vi "PPMS Monitor and Control.vi"() -> ()   [LabVIEW 2019, in "instrument.PPMS.lvclass"]
doc: "This VI will launch the PPMS 2 Instrument backend that will contunously monitor the state of the instrument and log to the DSC. The user has the option of launching a user interface (default) or allowing the backend to run headless. Run \"Launch PPMS2 UI.vi\" here or on a different computer to have a remote user interface. You can also use the APIs like \"Get Temperturature\" interact programmatically with the PPMS 2 Instrument backend."
uses:
  instrument.PPMS/instrument.PPMS.lvclass
  <vilib>/JKI/JKI SMO/SMO/Typedefs/SMOState --Enum.ctl
  <vilib>/JKI/JKI SMO/SMO.UI/Typedefs/SMO.UI State--enum.ctl
  C:/Program Files (x86)/National Instruments/LabVIEW 2019/user.lib/LevyLab/Instrument Framework/Instrument/Instrument.lvclass
  C:/Program Files (x86)/National Instruments/LabVIEW 2019/vi.lib/JKI/JKI SMO/SMO/SMO.lvclass
  instrument.PPMS UI/Instrument UI.PPMS.lvclass
  C:/Program Files (x86)/National Instruments/LabVIEW 2019/vi.lib/JKI/JKI SMO/SMO.UI/SMO.UI.lvclass
  C:/Program Files (x86)/National Instruments/LabVIEW 2019/user.lib/LevyLab/Instrument Framework/Instrument UI/Instrument UI.lvclass
  <userlib>/LevyLab/Configuration/Configuration.lvclass
  PPMS/Select PPMS--Enum.ctl
  <vilib>/Utility/sysdir.llb/System Directory Type.ctl
  <vilib>/JKI/JKI SMO/SMO/SMO.lvclass/SMO.ctl
  <vilib>/JKI/JKI SMO/SMO.UI/SMO.UI.lvclass/SMO.UI.ctl
  <vilib>/JKI/JKI SMO/SMO/Private/ReftoDVR--SMO.vi
  <vilib>/JKI/JKI SMO/SMO.UI/SMO.UI.ReftoDVR.vi
  <vilib>/JKI/JKI SMO/SMO/SMO.lvclass
  <vilib>/JKI/JKI SMO/SMO.UI/SMO.UI.lvclass
  <userlib>/LevyLab/Instrument Framework/Instrument UI/Instrument UI.lvclass
  PPMS/PPMS.lvlib
  <userlib>/LevyLab/Instrument Framework/Instrument/Instrument.lvclass
  <vilib>/Utility/config.llb/NI_LVConfig.lvlib
panel:
  in  "Examine Configuration.ini":bool
  out "version":string
  in  "Debug Mode":bool
  in  "Select PPMS":T1(ring) caption="Enum"
  in  "Stop Application":bool caption="Stop"
  in  "Start Application":bool caption="Play"
  in  "Splash Status":string="Push Start to Start..." caption="String"
  out "error out":errorcluster
  # "PPMS\nMonitor\n&\nControl"
  # "PPMS1: 130.49.180.18\nPPMS2: 130.49.180.87\nPPMS3: 130.49.180.47\nsimulate: localhost"
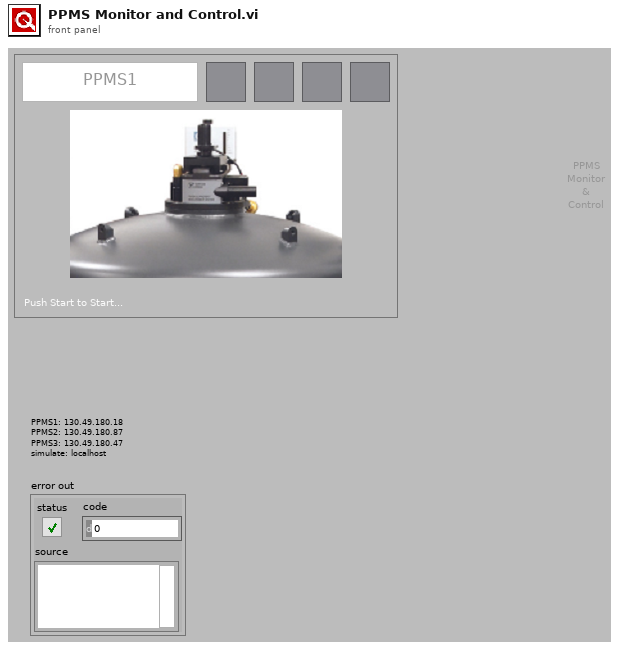
[diagram p1: front panel]
types:
  T1 = enum16{"PPMS1", "PPMS2", "PPMS3", "OptiCool", "PPMS-W-1", "Simulate PPMS", "Simulate DynaCool", "Simulate OptiCool"}
  T2 = typedef "SMO.lvclass/SMOState --Enum.ctl" = enum16{"unknown", "Created", "Started", "Stopped"}
  T3 = typedef "SMO.UI.lvclass/SMO.UI State--enum.ctl" = enum16{"unknown", "Opened", "Closed"}
  T4 = enum32{"Invalid", "Standard", "Closed", "Hidden", "Minimized", "Maximized"}
  T5 = enum32{"invalid app kind", "Development System", "Run Time System", "Student Edition", "Embedded LabVIEW", "Evaluation", "Custom"}
  T6 = typedef "PPMS.lvlib/Select PPMS--Enum.ctl" = enum16{"PPMS1", "PPMS2", "PPMS3", "OptiCool", "PPMS-W-1", "Simulate PPMS", "Simulate DynaCool", "Simulate OptiCool"}
  T7 = cluster{"Core":cluster{"Current VI Reference":refnum<vi>, "Close Panel on Exit?":bool}, "instrument.PPMS":refnum<class "instrument.PPMS.lvclass">, "Instrument UI.PPMS":refnum<class "Instrument UI.PPMS.lvclass">, "Select PPMS":T6, "Previous PPMS":T6, "UI Config":refnum<class "Configuration.lvclass">}
  T8 = cluster{"Current VI Reference":refnum<vi>, "Close Panel on Exit?":bool}
  T9 = typedef "System Directory Type.ctl" = i32
  T10 = typedef "NI_LVConfig.lvlib/Config Data RefNum.ctl" = refnum<k1>
  T11 = typedef "SMO.lvclass/Public Events.ctl" = cluster{"Error":refnum<user-event>, "State":refnum<user-event>, "Reserve State":refnum<user-event>}
  T12 = typedef "SMO.UI.lvclass/PublicEvents--Cluster.ctl" = cluster{"UI Hidden":refnum<user-event>, "UI State":refnum<user-event>}
  T13 = cluster{"Event Registration Refnum":refnum<event-registration>, "Event Registration Refnum":refnum<event-registration>}
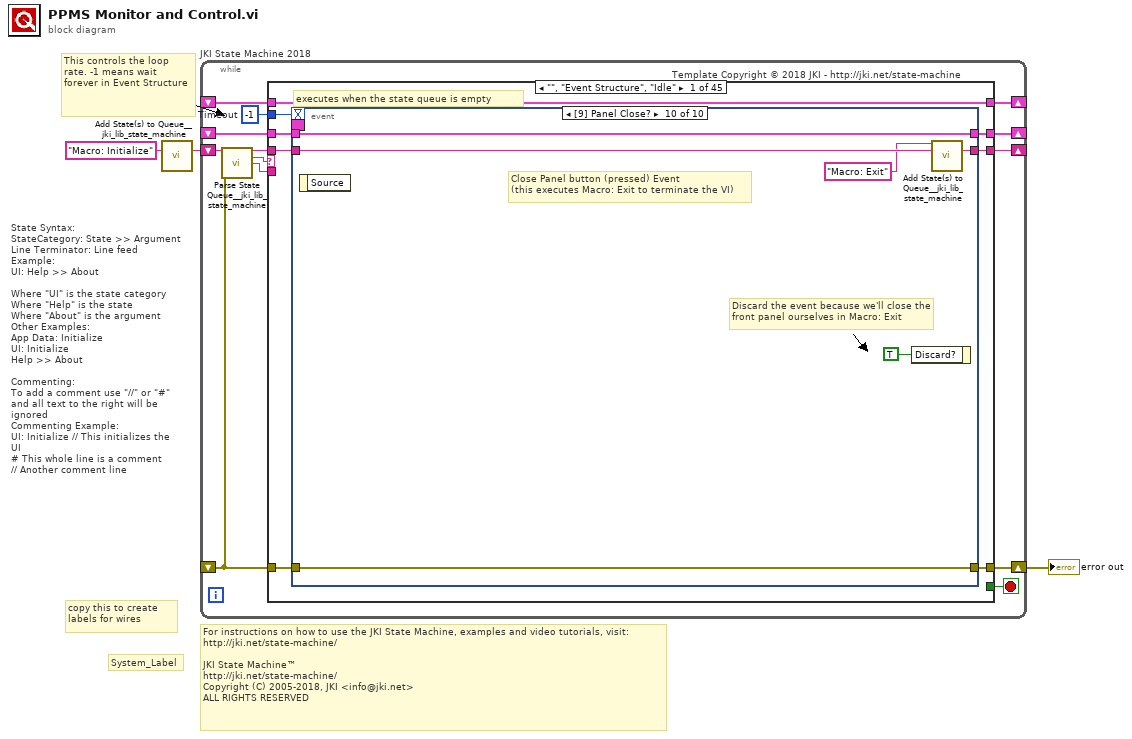
[diagram p0: block diagram]
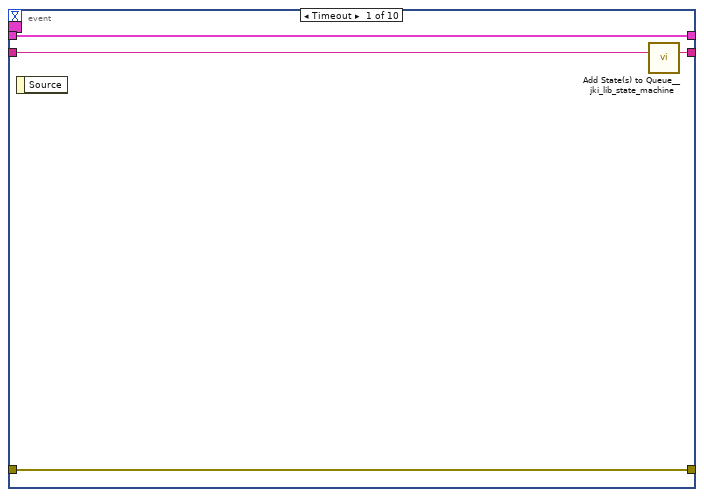
[diagram p2: hidden frame]
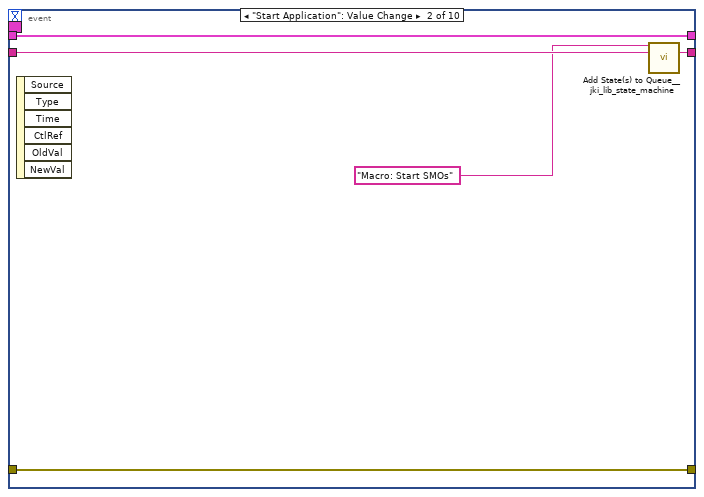
[diagram p3: hidden frame]
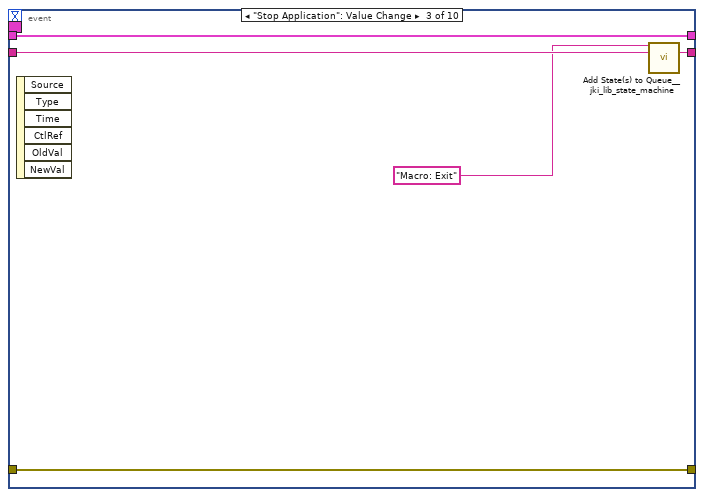
[diagram p4: hidden frame]
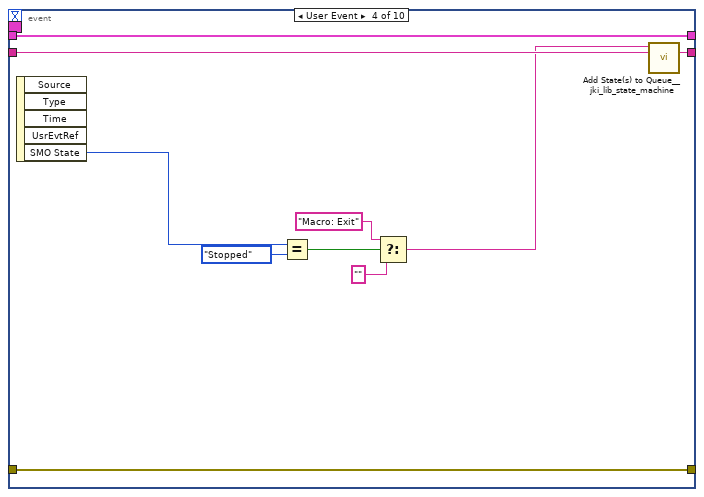
[diagram p5: hidden frame]
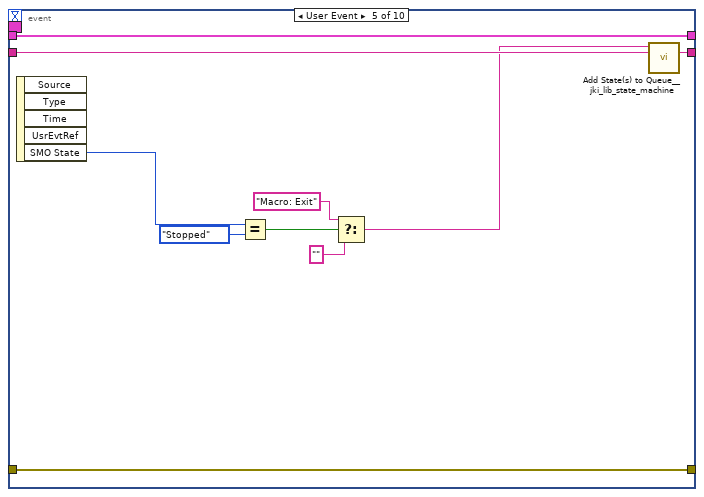
[diagram p6: hidden frame]
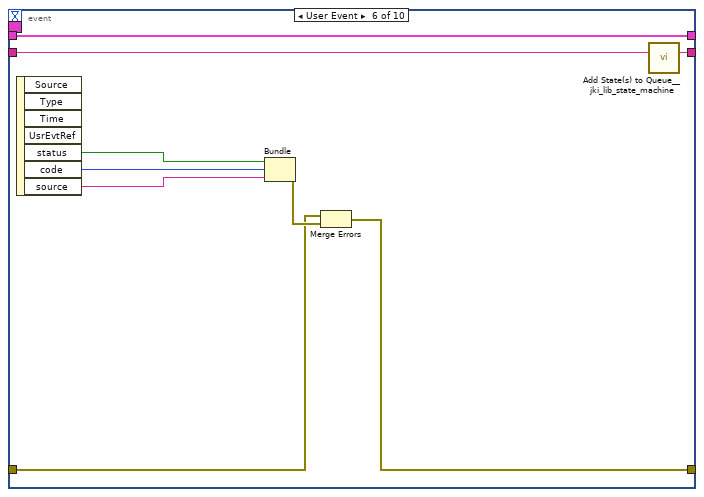
[diagram p7: hidden frame]
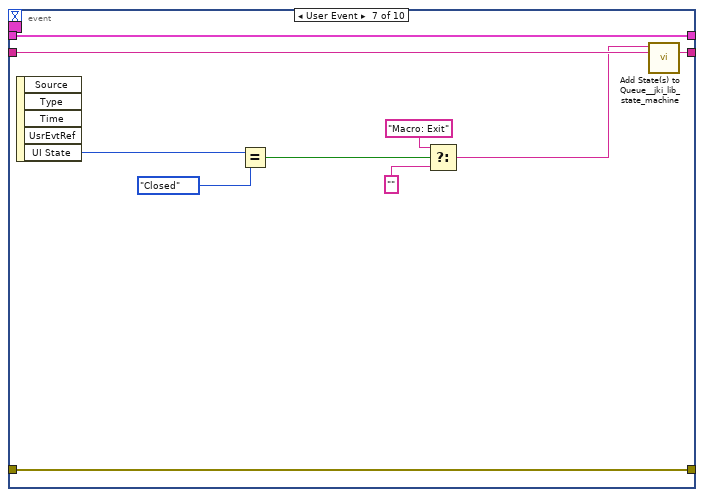
[diagram p8: hidden frame]
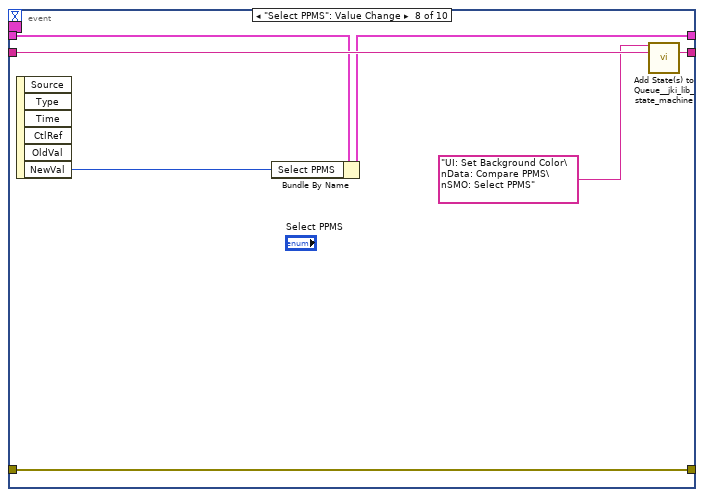
[diagram p9: hidden frame]
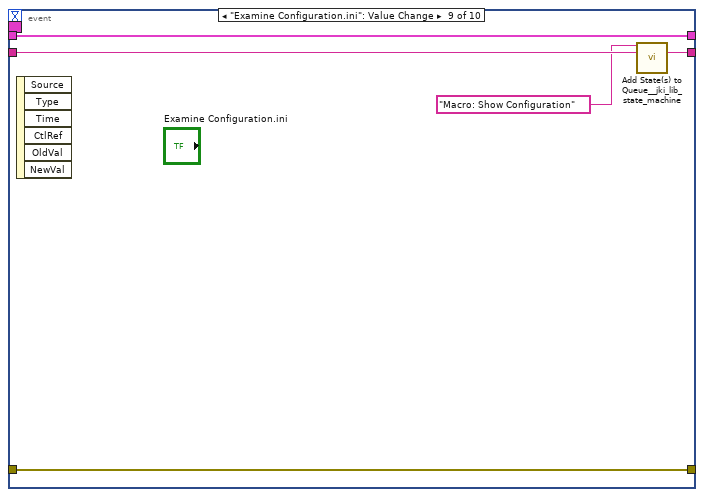
[diagram p10: hidden frame]
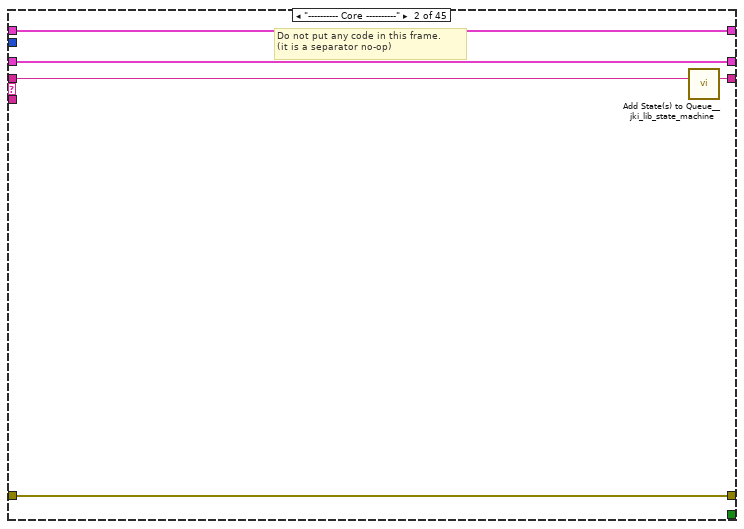
[diagram p11: hidden frame]
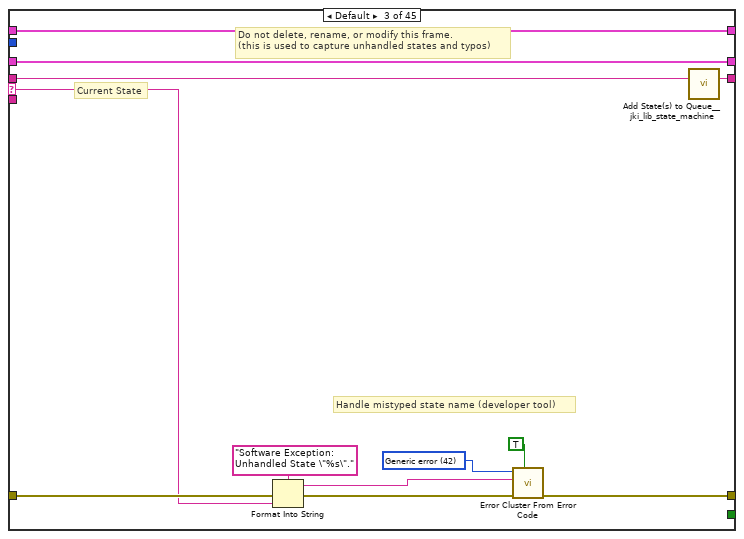
[diagram p12: hidden frame]
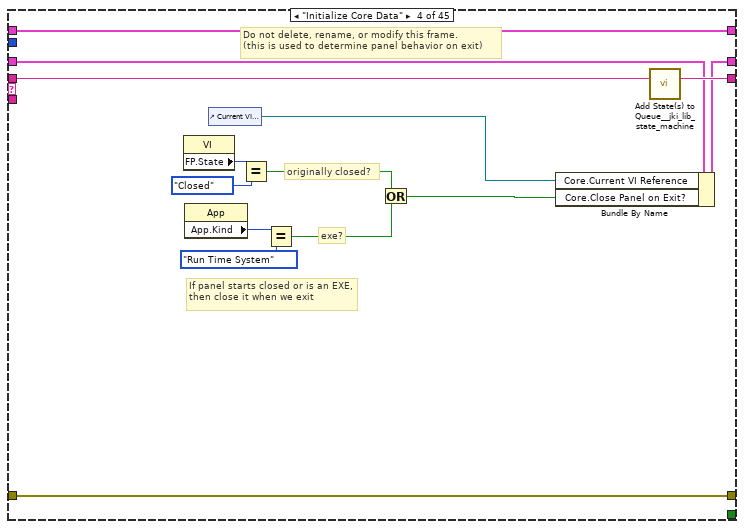
[diagram p13: hidden frame]
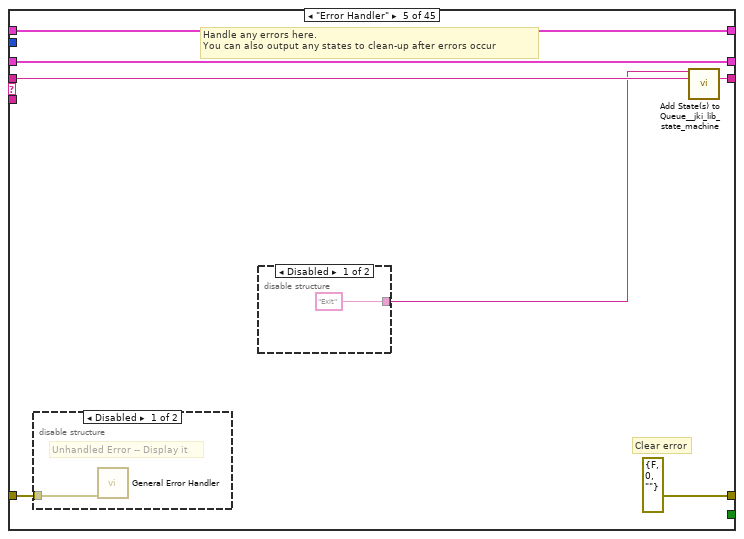
[diagram p14: hidden frame]
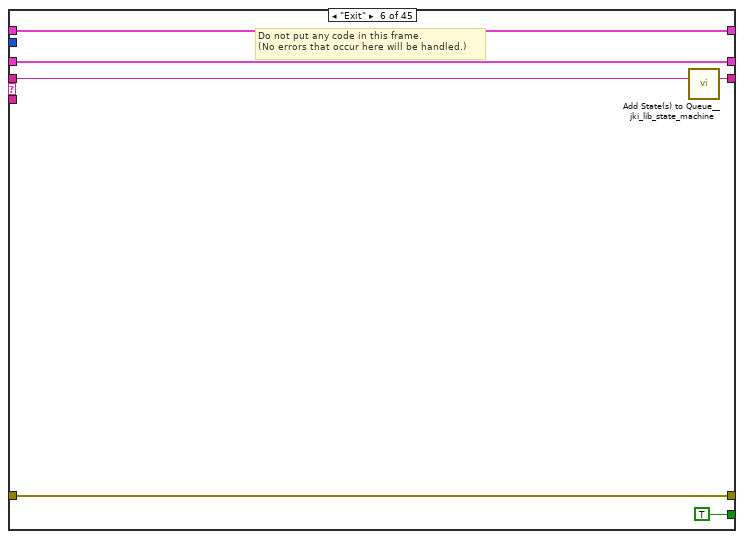
[diagram p17: hidden frame]
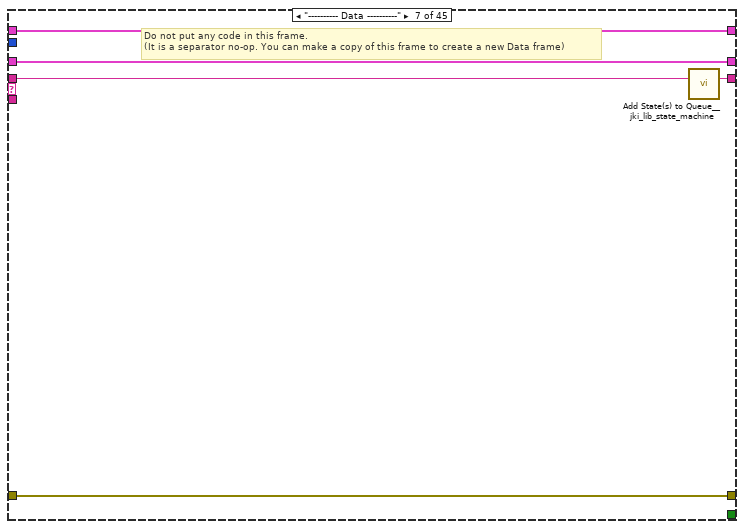
[diagram p18: hidden frame]
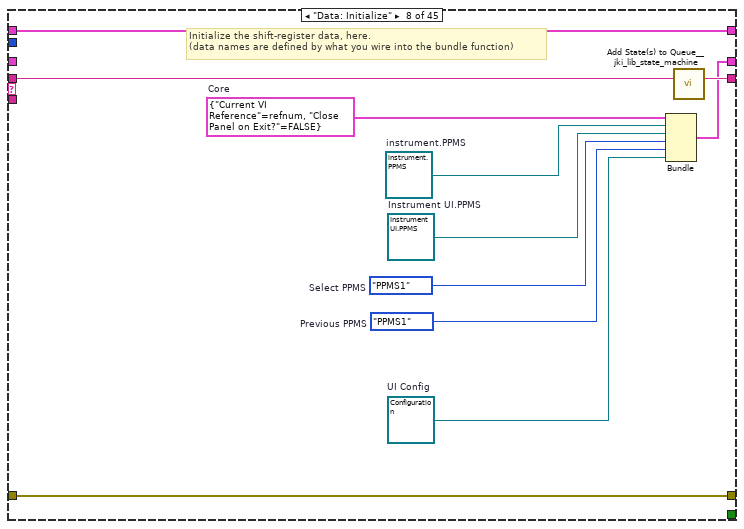
[diagram p19: hidden frame]
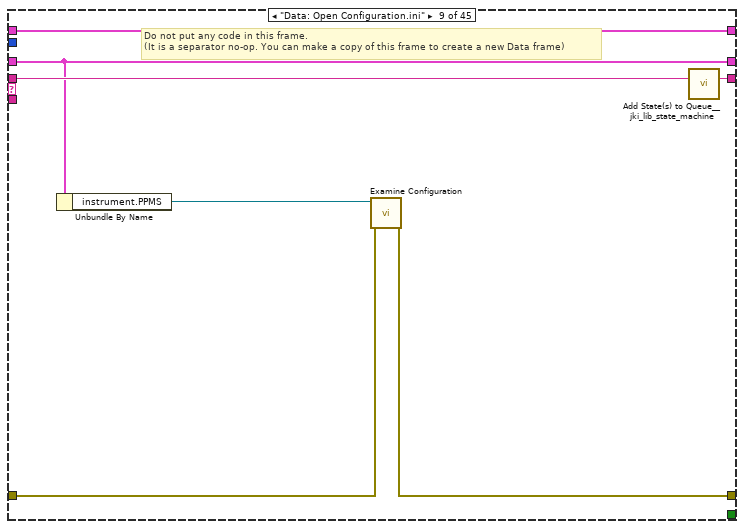
[diagram p20: hidden frame]
diagram:
  # "For instructions on how to use the JKI State Machine, examples and video tutorials, visit:\nhttp://jki.net/state-machine/\n\nJKI State Machine™\nhttp://jki.net/state-machine/\nCopyright (C) 2005-2018, JKI <info@jki.net>\nALL RIGHTS RESERVED"
  # "State Syntax:\nStateCategory: State >> Argument\nLine Terminator: Line feed\nExample:\nUI: Help >> About\n\nWhere \"UI\" is the state category\nWhere \"Help\" is the state\nWhere \"About\" is the argument\nOther Examples:\nApp Data: Initialize\nUI: Initialize\nHelp >> About\n\nCommenting:\nTo add a comment use \"//\" or \"#\" and all text to the right will be ignored\nCommenting Example:\nUI: Initialize // This initializes the UI\n# This whole line is a comment\n// Another comment line"
  # "copy this to create labels for wires"
  # "This controls the loop rate. -1 means wait forever in Event Structure"
  # "System_Label"
  n1 = call <vilib>:"Add State(s) to Queue__jki_lib_state_machine.vi"("State(s) in (\"\")"="Macro: Initialize") -> ("States Out"=w3:string)  [unwired: 14 in]
  n2 = while "JKI State Machine 2018" {
    shift-right: [w9] -> _
    shift-left: _ -> [w4]
    shift-right: [w12] -> w1
    shift-left: _ -> [w7]
    shift-right: [w11] -> _
    shift-left: w3 -> [w13]
    shift-right: [w6] -> _
    shift-left: _ -> [w5]
    stop <- w10 stop-if-true
    w8 = -1  # Timeout
    # "Template Copyright © 2018 JKI - http://jki.net/state-machine"
    n3 = call <vilib>:"Parse State Queue__jki_lib_state_machine.vi"("State Queue"=w13, "Error In (no error)"=w7) -> ("Remaining States"=w15:string, "Current State"=w16:string, "Arguments"=w14:string)  [unwired: 11 in]
    n4 = case shown="\"\", \"Event Structure\", \"Idle\"" w16 {
      selector: w16 -> [_ _ w102 _ _ _ _ _ _ _ _ _ _ _ _ _ _ _ _ _ _ _ _ _ _ _ _ _ _ _ _ _ _ _ _ _ _ _ _ _ _ _ _ _ _]
      tunnel: w15 -> [w24 w100 w106 w126 w133 w141 w146 w157 w164 w172 w179 w188 w214 w229 w235 w240 w250 w257 w269 w348 w361 w370 w382 w396 w401 w407 w413 w419 w425 w437 w442 w456 w467 w476 w487 w503 w517 w524 w535 w550 w565 w581 w590 w597 w602]
      tunnel: w14 -> [_ _ _ _ _ _ _ _ _ w165 _ _ _ _ _ _ _ w252 w263 _ _ _ _ _ _ _ _ _ _ _ _ _ _ _ _ _ _ _ _ _ _ _ _ w594 _]
      tunnel: [w21 w98 w108 w123 errorcluster {"status"=FALSE, "code"=0, "source"=""} ("error out") w138 w144 w154 w159 w170 w175 w181 w212 w218 w230 w238 w245 w253 w266 w338 w359 w363 w374 w387 w399 w405 w411 w417 w423 w435 w440 w449 w463 w468 w484 w499 w511 w518 w531 w546 w562 w578 w588 w592 w600] -> w12
      tunnel: w7 -> [w20 w98 w107 w123 w129 w138 w144 w154 w158 w170 w176 w180 w212 w220 w231 w238 w247 w254 w267 w339 w359 w364 w375 w389 w399 w405 w411 w417 w423 w435 w440 w444 w459 w469 w482 w495 w510 w519 w528 w543 w560 w574 w588 w593 w600]
      tunnel: [w23 w99 w105 w125 w132 w140 w145 w156 w163 w171 w178 w187 w213 w228 w234 w239 w249 w256 w268 w347 w360 w369 w381 w395 w400 w406 w412 w418 w424 w436 w441 w455 w466 w475 w486 w502 w516 w523 w534 w549 w564 w580 w589 w596 w601] -> w11
      tunnel: [_ _ _ _ _ TRUE _ _ _ _ _ _ _ _ _ _ _ _ _ _ _ _ _ _ _ _ _ _ _ _ _ _ _ _ _ _ _ _ _ _ _ _ _ _ _] -> w10
      tunnel: [w19 w97 w104 w124 w130 w139 w143 w155 w160 w169 w174 w185 w211 w223 w233 w237 w248 w255 w265 w336 w358 w366 w379 w393 w398 w404 w410 w416 w422 w434 w439 w453 w461 w471 w483 w500 w513 w521 w532 w547 w561 w577 w587 w595 w599] -> w9
      tunnel: w8 -> [w18 _ _ _ _ _ _ _ _ _ _ _ _ _ _ _ _ _ _ _ _ _ _ _ _ _ _ _ _ _ _ _ _ _ _ _ _ _ _ _ _ _ _ _ _]
      tunnel: [w17 w96 w101 w113 w127 w136 w142 w152 w162 w168 w173 w186 w210 w226 w232 w236 w246 w251 w262 w337 w357 w368 w380 w394 w397 w402 w408 w415 w421 w428 w438 w454 w465 w474 w485 w501 w515 w522 w533 w548 w563 w579 w586 w591 w598] -> w6
      tunnel: w5 -> [w17 w96 w101 w113 w127 w136 w142 w152 w162 w168 w173 w186 w210 _ w232 w236 w246 w251 w262 w337 w357 w368 w380 w394 w397 w402 w408 w415 w421 w428 w438 w454 w465 w474 w485 w501 w515 w522 w533 w548 w563 w579 w586 w591 w598]
      tunnel: w4 -> [w22 w97 w104 w119 w130 w139 w143 _ w160 w169 w174 w185 w211 w223 w233 w237 w248 w255 w265 w336 w358 w367 w377 w392 w398 w404 w410 w416 w422 w434 w439 w448 w460 w472 w483 w500 w514 w521 w532 w547 w561 w577 w587 w595 w599]
      frame "", "Event Structure", "Idle" {
        # "executes when the state queue is empty"
        n5 = event shown="[9] Panel Close?" {
          selector: w17 -> [_ _ _ _ _ _ _ _ _ _]
          dyn-events: _ -> [_ _ _ _ _ _ _ _ _ _]
          timeout: w18 -> [_ _ _ _ _ _ _ _ _ _]
          tunnel: w24 -> [w28 w33 w38 w48 w58 w67 w77 w84 w88 w95]
          tunnel: [w27 w32 w37 w47 w57 w66 w76 w83 w89 w94] -> w23
          tunnel: w22 -> [w25 w30 w35 w45 w55 w65 w75 w79 w85 w92]
          tunnel: [w26 w31 w36 w46 w56 w62 w74 w82 w86 w93] -> w21
          tunnel: w20 -> [w26 w31 w36 w46 w56 w63 w74 w82 w86 w93]
          tunnel: [w25 w30 w35 w45 w55 w65 w75 w78 w85 w92] -> w19
          event Timeout {
            n6 = event-data() -> ()  [unwired: 1 in, 1 out]
            n7 = call <vilib>:"Add State(s) to Queue__jki_lib_state_machine.vi"("State(s) in (\"\")"=w28) -> ("States Out"=w27:string)  [unwired: 14 in]
          }
          event "Start Application": Value Change {
            n8 = event-data() -> ()  [unwired: 1 in, 6 out]
            n9 = call <vilib>:"Add State(s) to Queue__jki_lib_state_machine.vi"("State(s) in Front (\"\")"="Macro: Start SMOs" ("State(s) in Front (\"\")"), "State(s) in (\"\")"=w33) -> ("States Out"=w32:string)  [unwired: 13 in]
          }
          event "Stop Application": Value Change {
            n10 = event-data() -> ()  [unwired: 1 in, 6 out]
            n11 = call <vilib>:"Add State(s) to Queue__jki_lib_state_machine.vi"("State(s) in Front (\"\")"="Macro: Exit" ("State(s) in Front (\"\")"), "State(s) in (\"\")"=w38) -> ("States Out"=w37:string)  [unwired: 13 in]
          }
          event User Event {
            n12 = event-data() -> ("SMO State"=w40:T2)  [unwired: 1 in, 4 out]
            n13 = Equal?(x=w40, y=SMOState_--Enum."Stopped") -> (x = y?=w43:bool)
            n14 = Select(t="Macro: Exit", s=w43, f="" ("State(s) in Front (\"\")")) -> (s? t:f=w39:string)
            n15 = call <vilib>:"Add State(s) to Queue__jki_lib_state_machine.vi"("State(s) in Front (\"\")"=w39, "State(s) in (\"\")"=w48) -> ("States Out"=w47:string)  [unwired: 13 in]
          }
          event User Event {
            n16 = event-data() -> ("SMO State"=w49:T2)  [unwired: 1 in, 4 out]
            n17 = Equal?(x=w49, y=SMOState_--Enum."Stopped") -> (x = y?=w53:bool)
            n18 = Select(t="Macro: Exit", s=w53, f="" ("State(s) in Front (\"\")")) -> (s? t:f=w51:string)
            n19 = call <vilib>:"Add State(s) to Queue__jki_lib_state_machine.vi"("State(s) in Front (\"\")"=w51, "State(s) in (\"\")"=w58) -> ("States Out"=w57:string)  [unwired: 13 in]
          }
          event User Event {
            n20 = event-data() -> ("status"=w59:bool, "code"=w61:i32, "source"=w60:string)  [unwired: 1 in, 4 out]
            n21 = Bundle("status"=w59, "code"=w61, "source"=w60) -> (w64:errorcluster)  [unwired: 1 in]
            n22 = Merge Errors(w63, w64) -> (w62:errorcluster)
            n23 = call <vilib>:"Add State(s) to Queue__jki_lib_state_machine.vi"("State(s) in (\"\")"=w67) -> ("States Out"=w66:string)  [unwired: 14 in]
          }
          event User Event {
            n24 = event-data() -> ("UI State"=w73:T3)  [unwired: 1 in, 4 out]
            n25 = Equal?(x=w73, y=SMO.UI_State--enum."Closed" ("UI State")) -> (x = y?=w71:bool)
            n26 = Select(t="Macro: Exit", s=w71, f="") -> (s? t:f=w68:string)
            n27 = call <vilib>:"Add State(s) to Queue__jki_lib_state_machine.vi"("State(s) in Front (\"\")"=w68, "State(s) in (\"\")"=w77) -> ("States Out"=w76:string)  [unwired: 13 in]
          }
          event "Select PPMS": Value Change {
            n28 = event-data() -> ("NewVal"=w80:T1)  [unwired: 1 in, 5 out]
            n29 = Bundle By Name(cluster=w79, "Select PPMS"=w80) -> (w78:T7)
            n30 = call <vilib>:"Add State(s) to Queue__jki_lib_state_machine.vi"("State(s) in Front (\"\")"="UI: Set Background Color\nData: Compare PPMS\nSMO: Select PPMS" ("State(s) in Front (\"\")"), "State(s) in (\"\")"=w84) -> ("States Out"=w83:string)  [unwired: 13 in]
          }
          event "Examine Configuration.ini": Value Change {
            n31 = event-data() -> ()  [unwired: 1 in, 6 out]
            n32 = call <vilib>:"Add State(s) to Queue__jki_lib_state_machine.vi"("State(s) in Front (\"\")"="Macro: Show Configuration" ("State(s) in Front (\"\")"), "State(s) in (\"\")"=w88) -> ("States Out"=w89:string)  [unwired: 13 in]
          }
          event Panel Close? {
            # "Discard the event because we'll close the front panel ourselves in Macro: Exit"
            # "Close Panel button (pressed) Event\n(this executes Macro: Exit to terminate the VI)"
            n33 = event-data() -> ()  [unwired: 1 in, 1 out]
            n34 = event-data("Discard?"=TRUE) -> ()  [unwired: 1 in, 1 out]
            n35 = call <vilib>:"Add State(s) to Queue__jki_lib_state_machine.vi"("State(s) in Front (\"\")"="Macro: Exit", "State(s) in (\"\")"=w95) -> ("States Out"=w94:string)  [unwired: 13 in]
          }
        }
      }
      frame "---------- Core ----------" {
        # "Do not put any code in this frame.\n(it is a separator no-op)"
        n36 = call <vilib>:"Add State(s) to Queue__jki_lib_state_machine.vi"("State(s) in (\"\")"=w100) -> ("States Out"=w99:string)  [unwired: 14 in]
      }
      frame Default {
        w111 = 42 items=["No error", "Argument error", "Memory is full", "Out of zone", "End of file", "File already open", "Generic file I/O error", "File not found", "File permission error", "Disk is full", "Duplicate path", "Too many files open", "System feature not enabled", "Resource file not found", "Cannot add resource", "Resource not found", "Image not found", "Image memory error", "Pen does not exist", "Config type invalid", "Config token not found", "Config parse error", "Config memory error", "Bad external code format", "Bad external code offset", "External code not present", "Null window", "Destroy window error", "Null menu", "Print aborted", "Bad print record", "Print driver error", "Windows error during printing", "Memory error during printing", "Print dialog error", "Generic print error", "Invalid device refnum", "Device not found", "Device parameter error", "Device unit error", "Cannot open device", "Device call aborted", "Generic error", "Cancelled by user", "Object ID too low", "Object ID too high", "Object not in heap", "Unknown heap", "Unknown object (invalid DefProc)", "Unknown object (DefProc not in table)", "Message out of range", "Invalid (null) method", "Unknown message", "Manager call not supported", "Bad address", "Network operation in progress", "Network operation timed out", "Connection is busy", "Network attribute not supported", "Network error", "Address in use", "System out of memory", "Connection aborted", "Connection refused", "Not connected", "Already connected", "Connection closed", "Initialization error (interapplication manager)", "Bad occurrence", "Wait on unbound occurrence handler", "Occurrence queue overflow", "Datalog type conflict", "Unused", "Unrecognized type (interapplication manager)", "Memory corrupt", "Failed to make temporary DLL", "Old CIN version", "Drag socket not found", "Failed to load drop-object", "Failed to register OLE object", "Failed to release OLE object", "Format specifier type mismatch", "Unknown format specifier", "Too few format specifiers", "Too many format specifiers", "Scan failed", "Newer CIN version", "Error converting to variant", "Runtime menu error", "Password tampered", "Variant attribute not found", "Incompatible variant data type", "Event data is not available", "Event Store is not present", "Occurrence is not found", "Event Queue is not created", "Event info is not available", "Refnum passed is NULL", "Error retrieving Class GUID", "Error retrieving CoClass GUID", "Error retrieving TypeLib GUID.", "Bad built application magic bytes.", "Specific driver is different from the specific driver associated with the Logical Name.", "There is no session opened to the class driver.", "Max Error", "MAX - Error with config objects", "MAX - Error loading configuration", "MAX - Group not supported"]
        # "Current State"
        # "Do not delete, rename, or modify this frame.\n(this is used to capture unhandled states and typos)"
        # "Handle mistyped state name (developer tool)"
        n37 = Format Into String(format string="Software Exception: Unhandled State \"%s\"." ("message"), error in=w107, w102) -> (resulting string=w110:string, error out=w109:errorcluster)  [unwired: 1 in]
        n38 = call <vilib>:"Error Cluster From Error Code.vi"("show call chain? (False)"=TRUE, "error in (no error)"=w109, "error message (\"\")"=w110, "error code (0)"=w111) -> ("error out"=w108:errorcluster)  [unwired: 5 in]
        n39 = call <vilib>:"Add State(s) to Queue__jki_lib_state_machine.vi"("State(s) in (\"\")"=w106) -> ("States Out"=w105:string)  [unwired: 14 in]
      }
      frame "Initialize Core Data" {
        # "Do not delete, rename, or modify this frame.\n(this is used to determine panel behavior on exit)"
        # "originally closed?"
        # "exe?"
        # "If panel starts closed or is an EXE, then close it when we exit"
        n40 = property class="VI"() -> ("FP.State"=w116:T4)  [unwired: 2 in, 2 out]
        n41 = property class="App"() -> ("App.Kind"=w122:T5)  [unwired: 2 in, 2 out]
        n42 = control-ref of="Current VI Reference"() -> (w117:refnum<vi>)
        n43 = Equal?(x=w116, y=T4."Closed" ("Front Panel Window:State")) -> (x = y?=w114:bool)
        n44 = Equal?(x=w122, y=T5."Run Time System" ("Application:Kind")) -> (x = y?=w120:bool)
        n45 = Or(x=w114, y=w120) -> (x .or. y?=w118:bool)
        n46 = Bundle By Name(cluster=w119, "Core.Current VI Reference"=w117, "Core.Close Panel on Exit?"=w118) -> (w124:T7)
        n47 = call <vilib>:"Add State(s) to Queue__jki_lib_state_machine.vi"("State(s) in (\"\")"=w126) -> ("States Out"=w125:string)  [unwired: 14 in]
      }
      frame "Error Handler" {
        # "Handle any errors here.\nYou can also output any states to clean-up after errors occur"
        # "Clear error"
        n48 = disable-structure shown="Disabled" {
          disable-tunnel: w129 -> [w135 _]
          frame Disabled {
            # "Unhandled Error -- Display it"
            n49 = call <vilib>:"General Error Handler.vi"("error in (no error)"=w135) -> ()  [unwired: 10 in, 5 out]
          }
          frame Enabled {
          }
        }
        n50 = disable-structure shown="Disabled" {
          disable-tunnel: ["Exit" _] -> w128
          frame Disabled {
          }
          frame Enabled {
          }
        }
        n51 = call <vilib>:"Add State(s) to Queue__jki_lib_state_machine.vi"("State(s) in Front (\"\")"=w128, "State(s) in (\"\")"=w133) -> ("States Out"=w132:string)  [unwired: 13 in]
      }
      frame "Exit" {
        # "Do not put any code in this frame.\n(No errors that occur here will be handled.)"
        n52 = call <vilib>:"Add State(s) to Queue__jki_lib_state_machine.vi"("State(s) in (\"\")"=w141) -> ("States Out"=w140:string)  [unwired: 14 in]
      }
      frame "---------- Data ----------" {
        # "Do not put any code in this frame.\n(It is a separator no-op. You can make a copy of this frame to create a new Data frame)"
        n53 = call <vilib>:"Add State(s) to Queue__jki_lib_state_machine.vi"("State(s) in (\"\")"=w146) -> ("States Out"=w145:string)  [unwired: 14 in]
      }
      frame "Data: Initialize" {
        w147 = Select_PPMS--Enum."PPMS1"  # Previous PPMS
        w148 = Select_PPMS--Enum."PPMS1"  # Select PPMS
        w149 = refnum<class "Configuration.lvclass"> refnum  # UI Config
        w150 = refnum<class "Instrument UI.PPMS.lvclass"> refnum  # Instrument UI.PPMS
        w151 = refnum<class "instrument.PPMS.lvclass"> refnum  # instrument.PPMS
        w153 = T8 {"Current VI Reference"=refnum, "Close Panel on Exit?"=FALSE}  # Core
        # "Initialize the shift-register data, here.\n(data names are defined by what you wire into the bundle function)"
        n54 = Bundle("Core"=w153, "instrument.PPMS"=w151, "Instrument UI.PPMS"=w150, "Select PPMS"=w148, "Previous PPMS"=w147, "UI Config"=w149) -> (w155:T7)  [unwired: 1 in]
        n55 = call <vilib>:"Add State(s) to Queue__jki_lib_state_machine.vi"("State(s) in (\"\")"=w157) -> ("States Out"=w156:string)  [unwired: 14 in]
      }
      frame "Data: Open Configuration.ini" {
        # "Do not put any code in this frame.\n(It is a separator no-op. You can make a copy of this frame to create a new Data frame)"
        n56 = Unbundle By Name(w160) -> ("instrument.PPMS"=w161:refnum<class "instrument.PPMS.lvclass">)
        n57 = call <userlib>:"Examine Configuration.vi"("error in (no error)"=w158, "Instrument in"=w161) -> ("error out"=w159:errorcluster)  [unwired: 8 in, 1 out]
        n58 = call <vilib>:"Add State(s) to Queue__jki_lib_state_machine.vi"("State(s) in (\"\")"=w164) -> ("States Out"=w163:string)  [unwired: 14 in]
      }
      frame "Data: Wait" {
        # "Do not put any code in this frame.\n(It is a separator no-op. You can make a copy of this frame to create a new Data frame)"
        n59 = Scan From String(input string=w165, default 1=u32 0) -> (output 1=w166:u32)  [unwired: 3 in, 3 out]
        n60 = Wait (ms)(milliseconds to wait=w166) -> ()  [unwired: 1 out]
        n61 = call <vilib>:"Add State(s) to Queue__jki_lib_state_machine.vi"("State(s) in (\"\")"=w172) -> ("States Out"=w171:string)  [unwired: 14 in]
      }
      frame "Data: Cleanup" {
        # "Cleanup any data and references, here.\n(this is called automatically, by the Macro: Exit)"
        n62 = Unbundle By Name(w174) -> ("Core.Current VI Reference"=w177:refnum<vi>)
        n63 = Close Reference(reference=w177, error in (no error)=w176) -> (error out=w175:errorcluster)
        n64 = call <vilib>:"Add State(s) to Queue__jki_lib_state_machine.vi"("State(s) in (\"\")"=w179) -> ("States Out"=w178:string)  [unwired: 14 in]
      }
      frame "Data: Compare PPMS" {
        # "Do not put any code in this frame.\n(It is a separator no-op. You can make a copy of this frame to create a new Data frame)"
        n65 = Unbundle By Name(w185) -> ("Select PPMS"=w184:T6, "Previous PPMS"=w183:T6)
        n66 = Not Equal?(x=w184, y=w183) -> (x != y?=w182:bool)
        n67 = case shown="True" w182 {
          tunnel: w180 -> [w189 w193]
          tunnel: [w189 w191] -> w181
          frame False {
            # "Selected matches previously selected (Do Nothing)"
          }
          frame True {
            w202 = T9 3 items=["User Home"=0, "User Desktop"=1, "User Documents"=2, "User Application Data"=3, "User Preferences"=4, "User Temporary"=5, "Public Documents"=6, "Public Application Data"=7, "Public Preferences"=8, "Public Cache"=13, "System Core Libraries"=9, "System Installed Libraries"=10, "Application Files"=11, "Boot Volume Root"=12] ("system directory type")
            # "Selected is different from previously selected (Clear Instrument section)\nThis is very inelegant but it should force the Insrtument subsection to create the proper PG log paths"
            n68 = call <vilib>:"Get System Directory.vi"("system directory type"=w202) -> ("system directory"=w201:path)  [unwired: 10 in]
            n69 = Build Path(base path=w201, name or relative path="LevyLab") -> (appended path=w200:path)
            n70 = Build Path(base path=w200, name or relative path="PPMS" ("Folder Name")) -> (appended path=w198:path)
            n71 = Build Path(base path=w198, name or relative path="configuration.ini") -> (appended path=w196:path)
            n72 = call <vilib>:"Open Config Data.vi"("error in (no error)"=w193, "create file if necessary (T)"=FALSE, "configuration file path"=w196) -> ("error out"=w192:errorcluster, "refnum"=w190:T10)  [unwired: 6 in, 1 out]
            n73 = case shown="No Error" w192 {
              selector: w192 -> [w207 _]
              tunnel: w190 -> [w208 _]
              tunnel: [w203 _] -> w191
              frame No Error {
                n74 = call <vilib>:"Remove Section.vi"("section"="Instrument", "error in (no error)"=w207, "refnum"=w208) -> ("error out"=w206:errorcluster, "section exists?"=w205:bool, "refnum out"=w204:T10)  [unwired: 6 in]
                n75 = call <vilib>:"Close Config Data.vi"("error in (no error)"=w206, "write file if changed (T)"=w205, "refnum"=w204) -> ("error out"=w203:errorcluster)  [unwired: 7 in, 1 out]
              }
              frame Error {
              }
            }
          }
        }
        n76 = call <vilib>:"Add State(s) to Queue__jki_lib_state_machine.vi"("State(s) in (\"\")"=w188) -> ("States Out"=w187:string)  [unwired: 14 in]
      }
      frame "---------- Events ----------" {
        # "Do not put any code in this frame.\n(It is a separator no-op. You can make a copy of this frame to create a new UI frame)"
        n77 = call <vilib>:"Add State(s) to Queue__jki_lib_state_machine.vi"("State(s) in (\"\")"=w214) -> ("States Out"=w213:string)  [unwired: 14 in]
      }
      frame "Events: Register" {
        # "Do not put any code in this frame.\n(It is a separator no-op. You can make a copy of this frame to create a new UI frame)"
        n78 = Unbundle By Name(w223) -> ("instrument.PPMS"=w222:refnum<class "instrument.PPMS.lvclass">, "Instrument UI.PPMS"=w221:refnum<class "Instrument UI.PPMS.lvclass">)
        n79 = call <vilib>:"GetPublicEvents.vi"("error in (no error)"=w220, "SMO"=w222) -> ("error out"=w219:errorcluster, "Public Events"=w224:T11)  [unwired: 7 in, 1 out]
        n80 = call <vilib>:"GetPublicEvents.vi"("error in (no error)"=w219, "SMO"=w221) -> ("error out"=w218:errorcluster, "Public Events"=w225:T11, "SMO out"=w216:refnum<class "Instrument UI.PPMS.lvclass">)  [unwired: 7 in]
        n81 = register-events(w224) -> (reference out=w227:refnum<event-registration>)  [unwired: 2 in, 1 out]
        n82 = call <vilib>:"SMO.UI.GetPublicEvents.vi"("SMO.UI"=w216) -> ("SMO.UI Public Events"=w215:T12)  [unwired: 8 in, 2 out]
        n83 = register-events(w225, w215) -> (reference out=w217:refnum<event-registration>)  [unwired: 2 in, 1 out]
        n84 = Bundle("Event Registration Refnum"=w227, "Event Registration Refnum"=w217) -> (w226:T13)  [unwired: 1 in]
        n85 = call <vilib>:"Add State(s) to Queue__jki_lib_state_machine.vi"("State(s) in (\"\")"=w229) -> ("States Out"=w228:string)  [unwired: 14 in]
      }
      frame "Events: Unregister" {
        # "Do not put any code in this frame.\n(It is a separator no-op. You can make a copy of this frame to create a new UI frame)"
        n86 = Unregister For Events(event registration refnum=w232, error in=w231) -> (error out=w230:errorcluster)
        n87 = call <vilib>:"Add State(s) to Queue__jki_lib_state_machine.vi"("State(s) in (\"\")"=w235) -> ("States Out"=w234:string)  [unwired: 14 in]
      }
      frame "---------- UI ----------" {
        # "Do not put any code in this frame.\n(It is a separator no-op. You can make a copy of this frame to create a new UI frame)"
        n88 = call <vilib>:"Add State(s) to Queue__jki_lib_state_machine.vi"("State(s) in (\"\")"=w240) -> ("States Out"=w239:string)  [unwired: 14 in]
      }
      frame "UI: Initialize" {
        # "Initialize the User Interface, here.\n(this is called automatically, by the Macro: Init)"
        n89 = invoke on="Stop Application" class="Bool" method="Reinit To Default"() -> ()  [unwired: 3 in, 3 out]
        n90 = invoke on="error out" class="Clust (strict)" method="Reinit To Default"() -> ()  [unwired: 3 in, 3 out]
        n91 = invoke on="Start Application" class="Bool" method="Reinit To Default"() -> ()  [unwired: 3 in, 3 out]
        n92 = call <userlib>:"Fit VI window to Largest Dec__ogtk.vi"("error in (no error)"=w247, "border spacing (2 px)"=0) -> ("error out"=w245:errorcluster)  [unwired: 4 in, 1 out]
        n93 = call <userlib>:"MGI Get Executable Version.vi"() -> ("Version"=w244:string)  [unwired: 7 in]
        n94 = Format Into String(format string="v%s", w244) -> (resulting string=→"version":string)  [unwired: 2 in, 1 out]
        n95 = call <vilib>:"Add State(s) to Queue__jki_lib_state_machine.vi"("State(s) in (\"\")"=w250) -> ("States Out"=w249:string)  [unwired: 14 in]
      }
      frame "UI: Cursor Set" {
        # "Argument"
        # "Set and Unset Cursor Busy.\n(Usage: \"UI: Cursor Set >> Busy|Idle\")"
        n96 = case shown="\"Busy\"" w252 {
          tunnel: w254 -> [w259 w261]
          tunnel: [w258 w260] -> w253
          frame "Idle", Default {
            n97 = call <vilib>:"Unset Busy.vi"("error in (no error)"=w259) -> ("error out"=w258:errorcluster)  [unwired: 10 in]
          }
          frame "Busy" {
            n98 = call <vilib>:"Set Busy.vi"("error in (no error)"=w261) -> ("error out"=w260:errorcluster)  [unwired: 9 in, 1 out]
          }
        }
        n99 = call <vilib>:"Add State(s) to Queue__jki_lib_state_machine.vi"("State(s) in (\"\")"=w257) -> ("States Out"=w256:string)  [unwired: 14 in]
      }
      frame "UI: Front Panel State" {
        # "Argument"
        # "Set Front Panel Open or Closed\n(Usage: \"UI: Front Panel State >> Open|Close\")"
        n100 = Unbundle By Name(w265) -> ("Core.Current VI Reference"=w264:refnum<vi>)
        n101 = case shown="\"Open\", \"Standard\", Default" w263 {
          tunnel: w267 -> [w275 w290 w301 w314 w327]
          tunnel: [w277 w291 w303 w316 w329] -> w266
          tunnel: w264 -> [w276 w288 w302 w315 w328]
          frame "Open", "Standard", Default {
            w270 = T4."Standard" ("State")
            n102 = property class="VI"(reference=w276, error in=w275) -> (reference out=w273:refnum<vi>, error out=w274:errorcluster, "FP.State"=w272:T4)
            n103 = Not Equal?(x=w272, y=w270) -> (x != y?=w271:bool)
            n104 = case shown="False" w271 {
              tunnel: [w281 w283] -> w277
              tunnel: w274 -> [w280 w283]
              tunnel: w273 -> [w279 _]
              tunnel: w270 -> [w278 _]
              frame True {
                n105 = invoke class="VI" method="FP.Open"(reference=w279, error in=w280, "Activate"=TRUE, "State"=w278) -> (error out=w281:errorcluster)  [unwired: 1 in, 4 out]
              }
              frame False {
              }
            }
          }
          frame "Close", "Closed" {
            n106 = property class="VI"(reference=w288, error in=w290) -> (reference out=w287:refnum<vi>, error out=w289:errorcluster, "FP.State"=w285:T4)
            n107 = Not Equal?(x=w285, y=T4."Closed" ("Front Panel Window:State")) -> (x != y?=w284:bool)
            n108 = case shown="True" w284 {
              tunnel: [w292 w295] -> w291
              tunnel: w289 -> [w292 w294]
              tunnel: w287 -> [_ w293]
              frame False {
              }
              frame True {
                n109 = invoke class="VI" method="FP.Close"(reference=w293, error in=w294) -> (error out=w295:errorcluster)  [unwired: 1 in, 2 out]
              }
            }
          }
          frame "Hidden", "Hide" {
            w296 = T4."Hidden" ("State")
            n110 = property class="VI"(reference=w302, error in=w301) -> (reference out=w299:refnum<vi>, error out=w300:errorcluster, "FP.State"=w298:T4)
            n111 = Not Equal?(x=w298, y=w296) -> (x != y?=w297:bool)
            n112 = case shown="True" w297 {
              tunnel: [w307 w308] -> w303
              tunnel: w300 -> [w306 w308]
              tunnel: w299 -> [w305 _]
              tunnel: w296 -> [w304 _]
              frame True {
                n113 = invoke class="VI" method="FP.Open"(reference=w305, error in=w306, "State"=w304) -> (error out=w307:errorcluster)  [unwired: 2 in, 4 out]
              }
              frame False {
              }
            }
          }
          frame "Minimize", "Minimized" {
            w309 = T4."Minimized" ("State")
            n114 = property class="VI"(reference=w315, error in=w314) -> (reference out=w312:refnum<vi>, error out=w313:errorcluster, "FP.State"=w311:T4)
            n115 = Not Equal?(x=w311, y=w309) -> (x != y?=w310:bool)
            n116 = case shown="True" w310 {
              tunnel: [w320 w321] -> w316
              tunnel: w313 -> [w319 w321]
              tunnel: w312 -> [w318 _]
              tunnel: w309 -> [w317 _]
              frame True {
                n117 = invoke class="VI" method="FP.Open"(reference=w318, error in=w319, "State"=w317) -> (error out=w320:errorcluster)  [unwired: 2 in, 4 out]
              }
              frame False {
              }
            }
          }
          frame "Maximize", "Maximized" {
            w322 = T4."Maximized" ("State")
            n118 = property class="VI"(reference=w328, error in=w327) -> (reference out=w325:refnum<vi>, error out=w326:errorcluster, "FP.State"=w324:T4)
            n119 = Not Equal?(x=w324, y=w322) -> (x != y?=w323:bool)
            n120 = case shown="True" w323 {
              tunnel: [w333 w334] -> w329
              tunnel: w326 -> [w332 w334]
              tunnel: w325 -> [w331 _]
              tunnel: w322 -> [w330 _]
              frame True {
                n121 = invoke class="VI" method="FP.Open"(reference=w331, error in=w332, "State"=w330) -> (error out=w333:errorcluster)  [unwired: 2 in, 4 out]
              }
              frame False {
              }
            }
          }
        }
        n122 = call <vilib>:"Add State(s) to Queue__jki_lib_state_machine.vi"("State(s) in (\"\")"=w269) -> ("States Out"=w268:string)  [unwired: 14 in]
      }
      frame "UI: Set Background Color" {
        # "Do not put any code in this frame.\n(It is a separator no-op. You can make a copy of this frame to create a new UI frame)"
        n123 = Unbundle By Name(w336) -> ("Select PPMS"=w335:T6)
        n124 = property class="VI"(error in=w339) -> (error out=w341:errorcluster, "Panel"=w342:refnum<vi>)  [unwired: 1 in, 1 out]
        n125 = case shown="\"Simulate DynaCool\"" w335 {
          tunnel: [u32 9077092 ("Color Box") u32 32639 ("Color Box") u32 6273022 ("Color Box") u32 16763690 ("Color Box") u32 16312751 ("Color Box") u32 16758979 ("Color Box") u32 12369084 ("Color Box") u32 16762248 ("Color Box")] -> w346
          frame "PPMS1" {
          }
          frame "PPMS2" {
          }
          frame "PPMS3" {
          }
          frame "OptiCool" {
          }
          frame "PPMS-W-1" {
          }
          frame "Simulate PPMS", Default {
          }
          frame "Simulate DynaCool" {
          }
          frame "Simulate OptiCool" {
          }
        }
        n126 = property class="Pnl"(reference=w342, error in=w341) -> (error out=w340:errorcluster, "Panes[]"=w343:refnum<vi>[])  [unwired: 1 out]
        n127 = Index Array(array=w343, index=0) -> (element=w345:refnum<vi>)
        n128 = property class="Pane"(reference=w345, error in=w340, "PaneColor"=w346) -> (error out=w338:errorcluster)  [unwired: 1 out]
        n129 = call <vilib>:"Add State(s) to Queue__jki_lib_state_machine.vi"("State(s) in (\"\")"=w348) -> ("States Out"=w347:string)  [unwired: 14 in]
      }
      frame "UI: Exit" {
        # "Do not put any code in this frame.\n(It is a separator no-op. You can make a copy of this frame to create a new UI frame)"
        n130 = invoke on="Start Application" class="Bool" method="Reinit To Default"() -> ()  [unwired: 3 in, 3 out]
        n131 = invoke on="Stop Application" class="Bool" method="Reinit To Default"() -> ()  [unwired: 3 in, 3 out]
        n132 = call <vilib>:"Add State(s) to Queue__jki_lib_state_machine.vi"("State(s) in (\"\")"=w361) -> ("States Out"=w360:string)  [unwired: 14 in]
      }
      frame "UI: Init UI Config" {
        # "Do not put any code in this frame.\n(It is a separator no-op. You can make a copy of this frame to create a new UI frame)"
        n133 = call <userlib>:"Default Path.vi"("error in (no error)"=w364, "Folder Name [Application Name]"="PPMS" ("Folder Name")) -> ("error out"=w363:errorcluster, "Configuration out"=w365:refnum<class "Configuration.lvclass">)  [unwired: 8 in]
        n134 = Bundle By Name(cluster=w367, "UI Config"=w365) -> (w366:T7)
        n135 = call <vilib>:"Add State(s) to Queue__jki_lib_state_machine.vi"("State(s) in (\"\")"=w370) -> ("States Out"=w369:string)  [unwired: 14 in]
      }
      frame "UI: Write UI Config" {
        w373 = cluster{"Select PPMS":T6} {"Select PPMS"=enum."PPMS3"}  # Launcher
        # "Do not put any code in this frame.\n(It is a separator no-op. You can make a copy of this frame to create a new UI frame)"
        n136 = Unbundle By Name(w377) -> ("UI Config"=w376:refnum<class "Configuration.lvclass">)
        n137 = local read "Select PPMS"() -> (w372:T1)
        n138 = Bundle By Name(cluster=w373, "Select PPMS"=w372) -> (w371:cluster{"Select PPMS":T6})
        n139 = call <userlib>:"Write Configuration.vi"("error in (no error)"=w375, "Variant"=w371, "Configuration in"=w376) -> ("error out"=w374:errorcluster, "Configuration out"=w378:refnum<class "Configuration.lvclass">)  [unwired: 7 in]
        n140 = Bundle By Name(cluster=w377, "UI Config"=w378) -> (w379:T7)
        n141 = call <vilib>:"Add State(s) to Queue__jki_lib_state_machine.vi"("State(s) in (\"\")"=w382) -> ("States Out"=w381:string)  [unwired: 14 in]
      }
      frame "UI: Read UI Config" {
        w385 = cluster{"Select PPMS":T6} {"Select PPMS"=enum."PPMS3"}  # Launcher
        # "Do not put any code in this frame.\n(It is a separator no-op. You can make a copy of this frame to create a new UI frame)"
        n142 = Unbundle By Name(w392) -> ("UI Config"=w391:refnum<class "Configuration.lvclass">)
        n143 = call <userlib>:"Read Configuration.vi"("INI Fomatted Cluster Type"=w385, "error in (no error)"=w389, "Configuration in"=w391) -> ("error out"=w388:errorcluster, "Configuration"=w386:variant, "Configuration out"=w390:refnum<class "Configuration.lvclass">)  [unwired: 6 in]
        n144 = Variant To Data(error in=w388, type=w385, Variant=w386) -> (data=w384:cluster{"Select PPMS":T6}, error out=w387:errorcluster)
        n145 = Unbundle(w384) -> ("Select PPMS"=w383:T6)
        n146 = property on="Select PPMS" class="Enum (strict)"("Val(Sgnl)"=w383) -> ()  [unwired: 2 in, 2 out]
        n147 = Bundle By Name(cluster=w392, "UI Config"=w390, "Select PPMS"=w383, "Previous PPMS"=w383) -> (w393:T7)
        n148 = call <vilib>:"Add State(s) to Queue__jki_lib_state_machine.vi"("State(s) in (\"\")"=w396) -> ("States Out"=w395:string)  [unwired: 14 in]
      }
      frame "---------- Macro ----------" {
        # "Do not put any code in this frame.\n(It is a separator no-op. You can make a copy of this frame to create a new Macro frame)"
        n149 = call <vilib>:"Add State(s) to Queue__jki_lib_state_machine.vi"("State(s) in (\"\")"=w401) -> ("States Out"=w400:string)  [unwired: 14 in]
      }
      frame "Macro: Initialize" {
        # "Initialization Macro\n(This is called once, when the VI starts)"
        n150 = call <vilib>:"Add State(s) to Queue__jki_lib_state_machine.vi"("State(s) in Front (\"\")"="Data: Initialize\nInitialize Core Data\n//Events: Register\nUI: Initialize\nUI: Front Panel State >> Open\nUI: Init UI Config\nUI: Read UI Config\nSplash: Set Status >> Push Start to Start...", "State(s) in (\"\")"=w407) -> ("States Out"=w406:string)  [unwired: 13 in]
      }
      frame "Macro: Show Configuration" {
        # "Initialization Macro\n(This is called once, when the VI starts)"
        n151 = call <vilib>:"Add State(s) to Queue__jki_lib_state_machine.vi"("State(s) in Front (\"\")"="Splash: Set Status >> Opening Configuration...\nData: Open Configuration.ini\nData: Wait >> 1000\nSplash: Set Status >> ...", "State(s) in (\"\")"=w413) -> ("States Out"=w412:string)  [unwired: 13 in]
      }
      frame "Macro: Start SMOs" {
        # "Do not put any code in this frame.\n(It is a separator no-op. You can make a copy of this frame to create a new Macro frame)"
        n152 = call <vilib>:"Add State(s) to Queue__jki_lib_state_machine.vi"("State(s) in Front (\"\")"="Splash: Set Status >> Creating Instrument...\nSMO: Create Instrument\nData: Wait >> 100\nSplash: Set Status >> Creating Instrument UI...\nSMO: Create Instrument UI\nData: Wait >> 100\nSplash: Set Status >> Registering Events...\nEvents: Register\nData: Wait >> 100\nSplash: Set Status >> Starting Instrument...\nSMO: Start Instrument\nData: Wait >> 100\nSplash: Set Status >> Instrument Process Started...\nData: Wait >> 100\nSplash: Set Status >> Starting User Interface...\nSMO: Start Instrument UI\nData: Wait >> 100\nUI: Front Panel State >> Hide\nSMO: Show Instrument UI" ("State(s) in Front (\"\")"), "State(s) in (\"\")"=w419) -> ("States Out"=w418:string)  [unwired: 13 in]
      }
      frame "Macro: Stop SMOs" {
        # "Do not put any code in this frame.\n(It is a separator no-op. You can make a copy of this frame to create a new Macro frame)"
        n153 = call <vilib>:"Add State(s) to Queue__jki_lib_state_machine.vi"("State(s) in Front (\"\")"="UI: Front Panel State >> Show\nSplash: Set Status >> Stopping Instrument...\nSMO: Stop Instrument\nData: Wait >> 100\nSplash: Set Status >> Destroying Instrument...\nSMO: Destroy Instrument\nData: Wait >> 100\nSplash: Set Status >>Hiding UI...\nSMO: Hide Instrument UI\nData: Wait >> 100\nSplash: Set Status >> Stopping UI...\nSMO: Stop Instrument UI\nData: Wait >> 100\nSplash: Set Status >> Destroying UI...\nSMO: Destroy Instrument UI" ("State(s) in Front (\"\")"), "State(s) in (\"\")"=w425) -> ("States Out"=w424:string)  [unwired: 13 in]
      }
      frame "Macro: Exit" {
        # "Exit Macro\n(This is called once, when the VI exits)"
        n154 = Unbundle By Name(w434) -> ("Core.Close Panel on Exit?"=w433:bool)
        n155 = Select(t="UI: Front Panel State >> Close", s=w433, f="") -> (s? t:f=w430:string)
        n156 = call <vilib>:"Add State(s) to Queue__jki_lib_state_machine.vi"("State(s) in Front (\"\")"="UI: Write UI Config\nUI: Front Panel State >> Open\nMacro: Stop SMOs\nUI: Exit", "State(s) in (\"\")"=w430, "State(s) at Back (\"\")"="Data: Cleanup\nEvents: Unregister\nExit") -> ("States Out"=w429:string)  [unwired: 12 in]
        n157 = call <vilib>:"Add State(s) to Queue__jki_lib_state_machine.vi"("State(s) in Front (\"\")"=w429, "State(s) in (\"\")"=w437) -> ("States Out"=w436:string)  [unwired: 13 in]
      }
      frame "---------- SMO ----------" {
        # "Do not put any code in this frame.\n(It is a separator no-op. You can make a copy of this frame to create a new Macro frame)"
        n158 = call <vilib>:"Add State(s) to Queue__jki_lib_state_machine.vi"("State(s) in (\"\")"=w442) -> ("States Out"=w441:string)  [unwired: 14 in]
      }
      frame "SMO: Create Instrument" {
        # "Do not put any code in this frame.\n(It is a separator no-op. You can make a copy of this frame to create a new Macro frame)"
        n159 = Unbundle By Name(w448) -> ("instrument.PPMS"=w447:refnum<class "instrument.PPMS.lvclass">)
        n160 = call "Get PPMS Class.vi"("error in (no error)"=w444, "instrument.PPMS"=w447) -> ("error out"=w445:errorcluster, "Select PPMS"=w443:T6, "instrument.PPMS out"=w446:refnum<class "instrument.PPMS.lvclass">)  [unwired: 7 in]
        n161 = case shown="\"Simulate PPMS\"..\"Simulate OptiCool\"" w443 {
          tunnel: [FALSE ("Configuration Window? [T]") TRUE ("Configuration Window? [T]")] -> w452
          frame "Simulate PPMS".."Simulate OptiCool" {
          }
          frame Default {
          }
        }
        n162 = call <userlib>:"Create Instrument SMO.vi"("error in (no error)"=w445, "Debug Mode? [F]"="Debug Mode", "Configuration Window? [T]"=w452, "Instrument in"=w446) -> ("error out"=w449:errorcluster, "Instrument out"=w450:refnum<class "instrument.PPMS.lvclass">)  [unwired: 6 in]
        n163 = Bundle By Name(cluster=w448, "instrument.PPMS"=w450) -> (w453:T7)
        n164 = call <vilib>:"Add State(s) to Queue__jki_lib_state_machine.vi"("State(s) in (\"\")"=w456) -> ("States Out"=w455:string)  [unwired: 14 in]
      }
      frame "SMO: Select PPMS" {
        # "Do not put any code in this frame.\n(It is a separator no-op. You can make a copy of this frame to create a new Macro frame)"
        n165 = local read "Select PPMS"() -> (w464:T1)
        n166 = call "Select PPMS Class.vi"("error in (no error)"=w459, "Select PPMS"=w464) -> ("error out"=w463:errorcluster, "instrument.PPMS out"=w462:refnum<class "instrument.PPMS.lvclass">)  [unwired: 8 in]
        n167 = Bundle By Name(cluster=w460, "instrument.PPMS"=w462) -> (w461:T7)
        n168 = call <vilib>:"Add State(s) to Queue__jki_lib_state_machine.vi"("State(s) in (\"\")"=w467) -> ("States Out"=w466:string)  [unwired: 14 in]
      }
      frame "SMO: Start Instrument" {
        # "Do not put any code in this frame.\n(It is a separator no-op. You can make a copy of this frame to create a new Macro frame)"
        n169 = Unbundle By Name(w472) -> ("instrument.PPMS"=w473:refnum<class "instrument.PPMS.lvclass">)
        n170 = call <vilib>:"Start.vi"("error in (no error)"=w469, "SMO"=w473) -> ("error out"=w468:errorcluster, "SMO out"=w470:refnum<class "instrument.PPMS.lvclass">)  [unwired: 8 in]
        n171 = Bundle By Name(cluster=w472, "instrument.PPMS"=w470) -> (w471:T7)
        n172 = call <vilib>:"Add State(s) to Queue__jki_lib_state_machine.vi"("State(s) in (\"\")"=w476) -> ("States Out"=w475:string)  [unwired: 14 in]
      }
      frame "SMO: Stop Instrument" {
        # "Do not put any code in this frame.\n(It is a separator no-op. You can make a copy of this frame to create a new Macro frame)"
        n173 = Unbundle By Name(w483) -> ("instrument.PPMS"=w478:refnum<class "instrument.PPMS.lvclass">)
        n174 = call <vilib>:"GetState.vi"("error in (no error)"=w482, "SMO"=w478) -> ("error out"=w481:errorcluster, "SMO State"=w479:T2, "SMO out"=w477:refnum<class "instrument.PPMS.lvclass">)  [unwired: 7 in]
        n175 = call <vilib>:"Clear Errors.vi"("error in (no error)"=w481) -> ("error out"=w480:errorcluster)  [unwired: 5 in, 1 out]
        n176 = case shown="\"Created\", \"Started\"" w479 {
          tunnel: [w488 w492] -> w484
          tunnel: w477 -> [_ w491]
          tunnel: w480 -> [w488 w490]
          frame Default {
          }
          frame "Created", "Started" {
            n177 = call <vilib>:"Stop.vi"("timeout in ms (-1)"=10000, "error in (no error)"=w490, "SMO"=w491) -> ("error out"=w492:errorcluster)  [unwired: 7 in, 1 out]
          }
        }
        n178 = call <vilib>:"Add State(s) to Queue__jki_lib_state_machine.vi"("State(s) in (\"\")"=w487) -> ("States Out"=w486:string)  [unwired: 14 in]
      }
      frame "SMO: Destroy Instrument" {
        # "Do not put any code in this frame.\n(It is a separator no-op. You can make a copy of this frame to create a new Macro frame)"
        n179 = Unbundle By Name(w500) -> ("instrument.PPMS"=w498:refnum<class "instrument.PPMS.lvclass">)
        n180 = call <vilib>:"GetState.vi"("error in (no error)"=w495, "SMO"=w498) -> ("error out"=w494:errorcluster, "SMO State"=w497:T2, "SMO out"=w493:refnum<class "instrument.PPMS.lvclass">)  [unwired: 7 in]
        n181 = call <vilib>:"Clear Errors.vi"("error in (no error)"=w494) -> ("error out"=w496:errorcluster)  [unwired: 5 in, 1 out]
        n182 = case shown="\"Stopped\"" w497 {
          tunnel: [w504 w507] -> w499
          tunnel: w496 -> [w504 w506]
          tunnel: w493 -> [_ w505]
          frame Default {
          }
          frame "Stopped" {
            n183 = call <vilib>:"Destroy.vi"("error in (no error)"=w506, "SMO"=w505) -> ("error out"=w507:errorcluster)  [unwired: 9 in]
          }
        }
        n184 = call <vilib>:"Add State(s) to Queue__jki_lib_state_machine.vi"("State(s) in (\"\")"=w503) -> ("States Out"=w502:string)  [unwired: 14 in]
      }
      frame "SMO: Create Instrument UI" {
        # "Do not put any code in this frame.\n(It is a separator no-op. You can make a copy of this frame to create a new Macro frame)"
        n185 = Unbundle By Name(w514) -> ("Instrument UI.PPMS"=w508:refnum<class "Instrument UI.PPMS.lvclass">, "instrument.PPMS"=w509:refnum<class "instrument.PPMS.lvclass">)
        n186 = call <userlib>:"Create UI.vi"("error in (no error)"=w510, "Instrument in"=w509, "Instrument UI"=w508) -> ("error out"=w511:errorcluster, "Instrument UI out"=w512:refnum<class "Instrument UI.PPMS.lvclass">)  [unwired: 7 in]
        n187 = Bundle By Name(cluster=w514, "Instrument UI.PPMS"=w512) -> (w513:T7)
        n188 = call <vilib>:"Add State(s) to Queue__jki_lib_state_machine.vi"("State(s) in (\"\")"=w517) -> ("States Out"=w516:string)  [unwired: 14 in]
      }
      frame "SMO: Start Instrument UI" {
        # "Do not put any code in this frame.\n(It is a separator no-op. You can make a copy of this frame to create a new Macro frame)"
        n189 = Unbundle By Name(w521) -> ("Instrument UI.PPMS"=w520:refnum<class "Instrument UI.PPMS.lvclass">)
        n190 = call <vilib>:"Start.vi"("error in (no error)"=w519, "SMO"=w520) -> ("error out"=w518:errorcluster)  [unwired: 8 in, 1 out]
        n191 = call <vilib>:"Add State(s) to Queue__jki_lib_state_machine.vi"("State(s) in (\"\")"=w524) -> ("States Out"=w523:string)  [unwired: 14 in]
      }
      frame "SMO: Show Instrument UI" {
        # "Do not put any code in this frame.\n(It is a separator no-op. You can make a copy of this frame to create a new Macro frame)"
        n192 = Unbundle By Name(w532) -> ("Instrument UI.PPMS"=w530:refnum<class "Instrument UI.PPMS.lvclass">)
        n193 = call <vilib>:"GetState.vi"("error in (no error)"=w528, "SMO"=w530) -> ("error out"=w526:errorcluster, "SMO State"=w525:T2, "SMO out"=w529:refnum<class "Instrument UI.PPMS.lvclass">)  [unwired: 7 in]
        n194 = call <vilib>:"Clear Errors.vi"("error in (no error)"=w526) -> ("error out"=w527:errorcluster)  [unwired: 5 in, 1 out]
        n195 = case shown="\"Started\"" w525 {
          tunnel: [w536 w539] -> w531
          tunnel: w529 -> [_ w538]
          tunnel: w527 -> [w536 w537]
          frame Default {
          }
          frame "Started" {
            n196 = call <vilib>:"Show.vi"("error in (no error)"=w537, "SMO.UI"=w538) -> ("error out"=w539:errorcluster)  [unwired: 8 in, 1 out]
          }
        }
        n197 = call <vilib>:"Add State(s) to Queue__jki_lib_state_machine.vi"("State(s) in (\"\")"=w535) -> ("States Out"=w534:string)  [unwired: 14 in]
      }
      frame "SMO: Hide Instrument UI" {
        # "Do not put any code in this frame.\n(It is a separator no-op. You can make a copy of this frame to create a new Macro frame)"
        n198 = Unbundle By Name(w547) -> ("Instrument UI.PPMS"=w545:refnum<class "Instrument UI.PPMS.lvclass">)
        n199 = call <vilib>:"GetState.vi"("error in (no error)"=w543, "SMO"=w545) -> ("error out"=w541:errorcluster, "SMO State"=w540:T2, "SMO out"=w544:refnum<class "Instrument UI.PPMS.lvclass">)  [unwired: 7 in]
        n200 = call <vilib>:"Clear Errors.vi"("error in (no error)"=w541) -> ("error out"=w542:errorcluster)  [unwired: 5 in, 1 out]
        n201 = case shown="\"Started\"" w540 {
          tunnel: [w551 w554] -> w546
          tunnel: w544 -> [_ w553]
          tunnel: w542 -> [w551 w552]
          frame Default {
          }
          frame "Started" {
            n202 = call <vilib>:"Hide.vi"("error in (no error)"=w552, "SMO.UI"=w553) -> ("error out"=w554:errorcluster)  [unwired: 8 in, 1 out]
          }
        }
        n203 = call <vilib>:"Add State(s) to Queue__jki_lib_state_machine.vi"("State(s) in (\"\")"=w550) -> ("States Out"=w549:string)  [unwired: 14 in]
      }
      frame "SMO: Stop Instrument UI" {
        # "Do not put any code in this frame.\n(It is a separator no-op. You can make a copy of this frame to create a new Macro frame)"
        n204 = Unbundle By Name(w561) -> ("Instrument UI.PPMS"=w556:refnum<class "Instrument UI.PPMS.lvclass">)
        n205 = call <vilib>:"GetState.vi"("error in (no error)"=w560, "SMO"=w556) -> ("error out"=w559:errorcluster, "SMO State"=w557:T2, "SMO out"=w555:refnum<class "Instrument UI.PPMS.lvclass">)  [unwired: 7 in]
        n206 = call <vilib>:"Clear Errors.vi"("error in (no error)"=w559) -> ("error out"=w558:errorcluster)  [unwired: 5 in, 1 out]
        n207 = case shown="\"Created\", \"Started\"" w557 {
          tunnel: [w566 w570] -> w562
          tunnel: w555 -> [_ w569]
          tunnel: w558 -> [w566 w568]
          frame Default {
          }
          frame "Created", "Started" {
            n208 = call <vilib>:"Stop.vi"("timeout in ms (-1)"=5000, "error in (no error)"=w568, "SMO"=w569) -> ("error out"=w570:errorcluster)  [unwired: 7 in, 1 out]
          }
        }
        n209 = call <vilib>:"Add State(s) to Queue__jki_lib_state_machine.vi"("State(s) in (\"\")"=w565) -> ("States Out"=w564:string)  [unwired: 14 in]
      }
      frame "SMO: Destroy Instrument UI" {
        # "Do not put any code in this frame.\n(It is a separator no-op. You can make a copy of this frame to create a new Macro frame)"
        n210 = Unbundle By Name(w577) -> ("Instrument UI.PPMS"=w576:refnum<class "Instrument UI.PPMS.lvclass">)
        n211 = call <vilib>:"GetState.vi"("error in (no error)"=w574, "SMO"=w576) -> ("error out"=w573:errorcluster, "SMO State"=w571:T2, "SMO out"=w575:refnum<class "Instrument UI.PPMS.lvclass">)  [unwired: 7 in]
        n212 = call <vilib>:"Clear Errors.vi"("error in (no error)"=w573) -> ("error out"=w572:errorcluster)  [unwired: 5 in, 1 out]
        n213 = case shown="\"Stopped\"" w571 {
          tunnel: w572 -> [w582 w585]
          tunnel: [w582 w584] -> w578
          tunnel: w575 -> [_ w583]
          frame Default {
          }
          frame "Stopped" {
            n214 = call <vilib>:"Destroy.vi"("error in (no error)"=w585, "SMO"=w583) -> ("error out"=w584:errorcluster)  [unwired: 9 in]
          }
        }
        n215 = call <vilib>:"Add State(s) to Queue__jki_lib_state_machine.vi"("State(s) in (\"\")"=w581) -> ("States Out"=w580:string)  [unwired: 14 in]
      }
      frame "---------- Splash ----------" {
        # "Template Separator\n(You can make a copy of, or modify, this frame)"
        n216 = call <vilib>:"Add State(s) to Queue__jki_lib_state_machine.vi"("State(s) in (\"\")"=w590) -> ("States Out"=w589:string)  [unwired: 14 in]
      }
      frame "Splash: Set Status" {
        # "Your code here.\n(You can make a copy of, or modify, this frame)"
        n217 = property on="Splash Status" class="Str"(error in=w593, "Value"=w594) -> (error out=w592:errorcluster)  [unwired: 1 in, 1 out]
        n218 = call <vilib>:"Add State(s) to Queue__jki_lib_state_machine.vi"("State(s) in (\"\")"=w597) -> ("States Out"=w596:string)  [unwired: 14 in]
      }
      frame "Splash: 2" {
        # "Your code here.\n(You can make a copy of, or modify, this frame)"
        n219 = call <vilib>:"Add State(s) to Queue__jki_lib_state_machine.vi"("State(s) in (\"\")"=w602) -> ("States Out"=w601:string)  [unwired: 14 in]
      }
    }
  }
  "error out" <- w1
